vi "Stim prot to numeric array.vi"(9 "Calibration Key":string, 10 "Skip Pixel Mapping? (Same I/S Path)":bool, 11 "Stm Protocol":string[][](array[string])=[["1[73,55]", " 50u", " 50u", " 1", " 0", " 50u"], ["2[118,83]", " 50u", " 50u", " 1", " 0", " 50u"], ["3[102,121]", " 50u", " 50u", " 1", " 0", " 50u"], ["4[74,129]", " 50u", " 50u", " 1", " 0", " 50u"], ["5[83,156]", " 50u", " 50u", " 1", " 0", " 50u"]]) -> (1 "Stim Array (with voltage) OUT":T1[](array[typedef]))   [LabVIEW 2012]
uses:
  Custom Controls and Typedefs/Stim Waveform Parameters.ctl
  Custom Controls and Typedefs/Params for Galvo Voltage Calculation (Y Axis).ctl
  Custom Controls and Typedefs/Params for Galvo Voltage Calculation (X Axis).ctl
  GFG/GFG library.lvlib
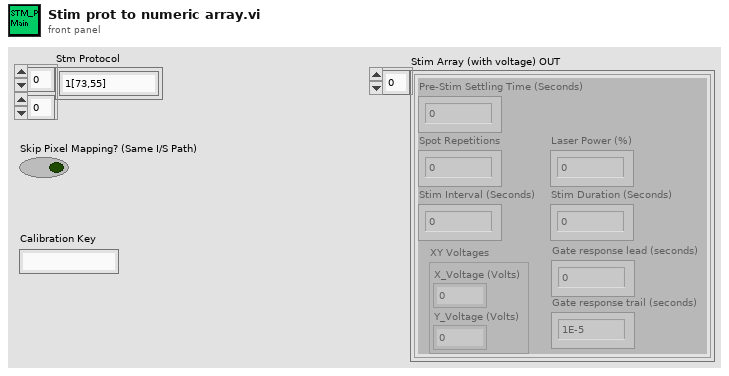
[diagram p1: front panel]
types:
  T1 = typedef "Stim Waveform Parameters.ctl" = cluster{"Stim Interval (Seconds)":dbl, "Pre-Stim Settling Time (Seconds)":dbl, "Stim Duration (Seconds)":dbl, "Spot Repetitions":i32, "Laser Power (%)":dbl, "XY Voltages":cluster{"X_Voltage (Volts)":dbl, "Y_Voltage (Volts)":dbl}, "Gate response lead (seconds)":dbl, "Gate response trail (seconds)":dbl}
  T2 = typedef "Params for Galvo Voltage Calculation (X Axis).ctl" = cluster{"X.Voltage(Max)":dbl, "X.Volt.Offset":dbl, "Tot.X.Pixels":u32, "X.Pixel.Index":u32}
  T3 = typedef "Params for Galvo Voltage Calculation (Y Axis).ctl" = cluster{"Y.Voltage(Max)":dbl, "Y.Volt.Offset":dbl, "Tot.Y.Pixels":u32, "Y.Pixel.Index":u32}
  T4 = typedef "Calibration Key Param structure.ctl" = cluster{"GFG Variable Name":string, "Data Type":T5, "Value":variant}
  T5 = typedef "VariantType.lvlib/Type.ctl" = enum8{"Invalid Type", "Void", "I8", "I16", "I32", "I64", "U8", "U16", "U32", "U64", "Single Float", "Double Float", "Extended Float", "Single Complex", "Double Complex", "Extended Complex", "Enum U8", "Enum U16", "Enum U32", "Enum U64", "Single Float With Unit", "Double Float With Unit", "Extended Float With Unit", "Single Complex with Unit", "Double Complex with Unit", "Extended Complex with Unit", "Boolean", "String", "Path", "Picture", "Tag", "Array", "Cluster", "Variant", "LV Variant", "Waveform", "Timestamp", "Digital Waveform", "Digital Data", "ExpressData", "Refnum", "External Data", "VI", "Poly VI", "LabVIEW Class Instance", "Fixed Point"}
  T6 = cluster{"X_Pixel_Voltage":dbl, "Y_Pixel_Voltage":dbl}
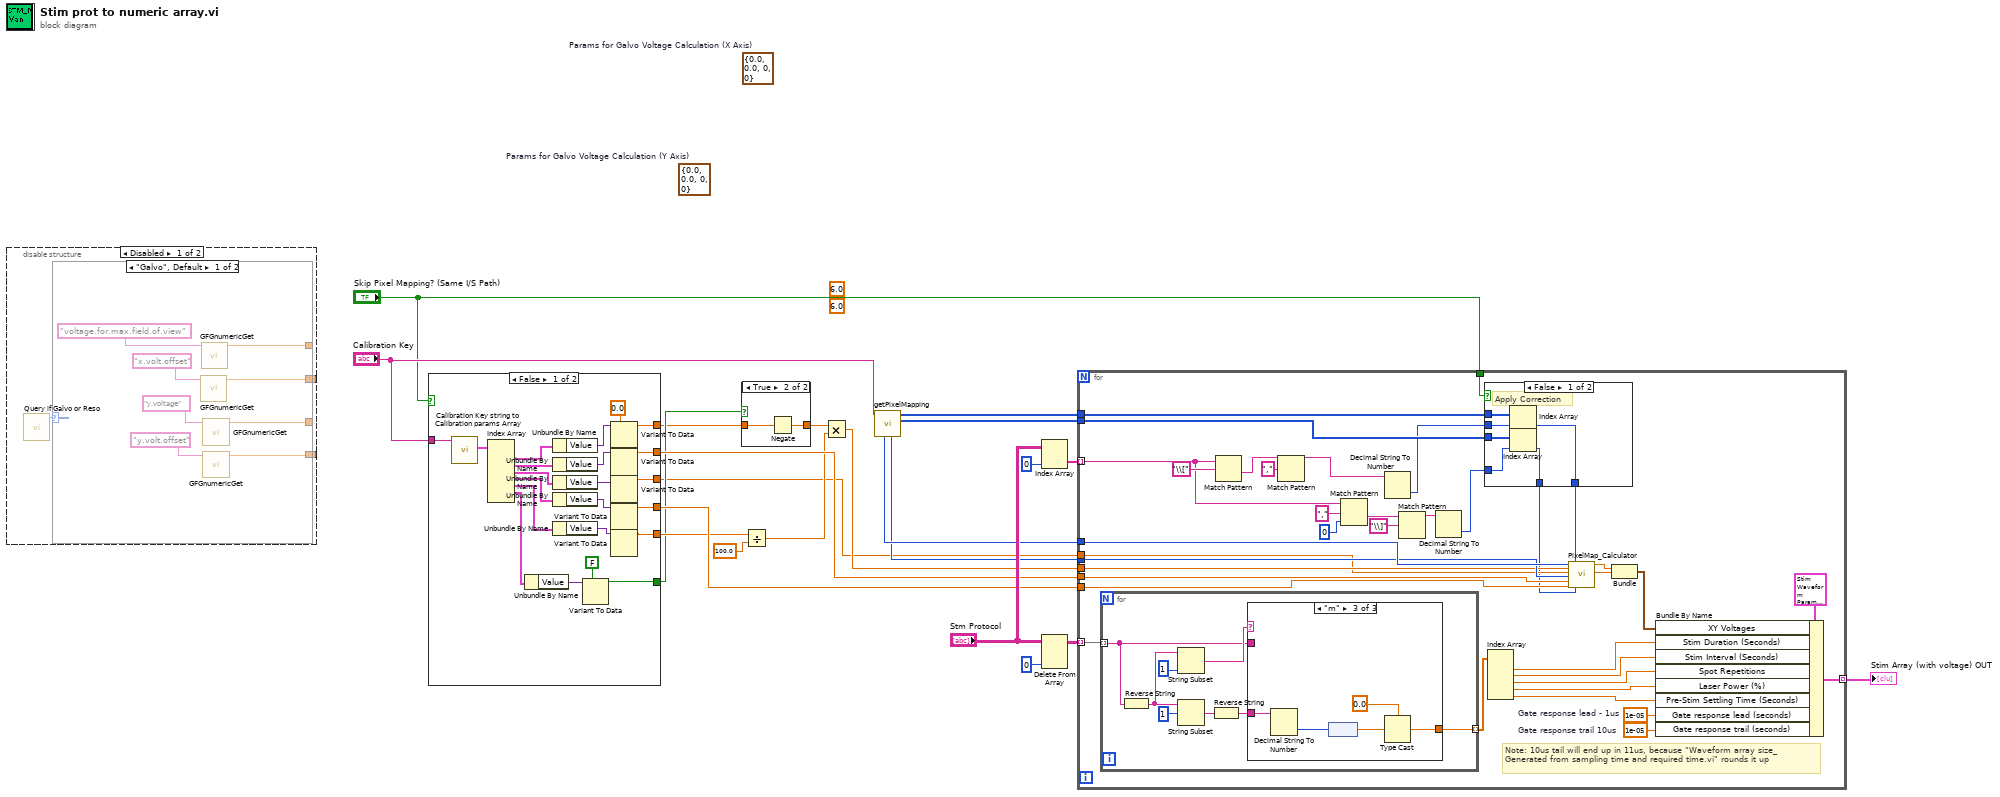
[diagram p0: block diagram]
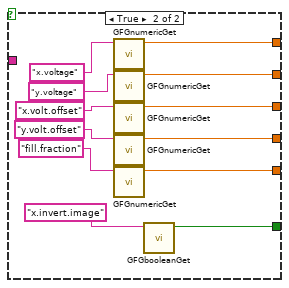
[diagram p3: hidden frame]
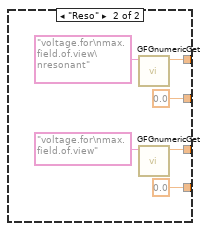
[diagram p4: hidden frame]
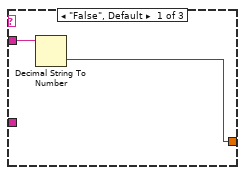
[diagram p7: hidden frame]
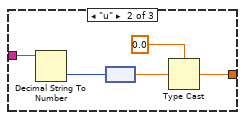
[diagram p8: hidden frame]
diagram:
  (unwired) T2 {"X.Voltage(Max)"=0.0, "X.Volt.Offset"=0.0, "Tot.X.Pixels"=0, "X.Pixel.Index"=0}  # Params for Galvo Voltage Calculation (X Axis)
  (unwired) T3 {"Y.Voltage(Max)"=0.0, "Y.Volt.Offset"=0.0, "Tot.Y.Pixels"=0, "Y.Pixel.Index"=0}  # Params for Galvo Voltage Calculation (Y Axis)
  (unwired) 6.0 ("Numeric")
  (unwired) 6.0 ("Numeric")
  n1 = disable-structure shown="Disabled" {
    disable-tunnel: [w24 _] -> _
    disable-tunnel: [w23 _] -> _
    frame Disabled {
      n2 = call "Query if Galvo or Reso.vi"() -> ("System Type"=w25:enum16{"Galvo", "Reso"})  [unwired: 10 in, 1 out]
      n3 = case shown="\"Galvo\", Default" w25 {
        tunnel: [w29 w37] -> _
        tunnel: [w28 0.0 ("Numeric")] -> w24
        tunnel: [w27 w36] -> _
        tunnel: [w26 0.0 ("Numeric")] -> w23
        frame "Galvo", Default {
          n4 = call "GFGnumericGet.vi"("Variable Name in"="x.volt.offset") -> ("Numeric"=w28:dbl)  [unwired: 8 in, 2 out]
          n5 = call "GFGnumericGet.vi"("Variable Name in"="voltage.for.max.field.of.view") -> ("Numeric"=w29:dbl)  [unwired: 8 in, 2 out]
          n6 = call "GFGnumericGet.vi"("Variable Name in"="y.voltage") -> ("Numeric"=w27:dbl)  [unwired: 8 in, 2 out]
          n7 = call "GFGnumericGet.vi"("Variable Name in"="y.volt.offset") -> ("Numeric"=w26:dbl)  [unwired: 8 in, 2 out]
        }
        frame "Reso" {
          n8 = call "GFGnumericGet.vi"("Variable Name in"="voltage.for\nmax.field.of.view\nresonant") -> ("Numeric"=w37:dbl)  [unwired: 8 in, 2 out]
          n9 = call "GFGnumericGet.vi"("Variable Name in"="voltage.for\nmax.field.of.view") -> ("Numeric"=w36:dbl)  [unwired: 8 in, 2 out]
        }
      }
    }
    frame Enabled {
    }
  }
  n10 = case shown="False" "Skip Pixel Mapping? (Same I/S Path)" {
    tunnel: "Calibration Key" -> [w61 _]
    tunnel: [w40 w66] -> w3
    tunnel: [w51 w67] -> w11
    tunnel: [w50 w65] -> w10
    tunnel: [w46 w64] -> w9
    tunnel: [w45 w68] -> w2
    tunnel: [w41 w62] -> w4
    frame False {
      w47 = 0.0
      n11 = call "Calibration Key string to Calibration params Array.vi"("Key String IN"=w61) -> ("Photostim Galvo Key Array"=w60:T4[])  [unwired: 8 in, 2 out]
      n12 = Index Array(array=w60) -> (element #1=w59:T4, element #2=w58:T4, element #3=w57:T4, element #4=w56:T4, element #5=w49:T4, element #6=w43:T4)  [unwired: 7 in, 1 out]
      n13 = Unbundle By Name(w43) -> ("Value"=w44:variant)
      n14 = Unbundle By Name(w59) -> ("Value"=w55:variant)
      n15 = Unbundle By Name(w58) -> ("Value"=w54:variant)
      n16 = Unbundle By Name(w57) -> ("Value"=w53:variant)
      n17 = Unbundle By Name(w56) -> ("Value"=w52:variant)
      n18 = Unbundle By Name(w49) -> ("Value"=w48:variant)
      n19 = Variant To Data(type=FALSE, Variant=w44) -> (data=w41:bool)  [unwired: 1 in, 1 out]
      n20 = Variant To Data(type=w47, Variant=w55) -> (data=w45:dbl)  [unwired: 1 in, 1 out]
      n21 = Variant To Data(type=w47, Variant=w54) -> (data=w51:dbl)  [unwired: 1 in, 1 out]
      n22 = Variant To Data(type=w47, Variant=w53) -> (data=w40:dbl)  [unwired: 1 in, 1 out]
      n23 = Variant To Data(type=w47, Variant=w52) -> (data=w50:dbl)  [unwired: 1 in, 1 out]
      n24 = Variant To Data(type=w47, Variant=w48) -> (data=w46:dbl)  [unwired: 1 in, 1 out]
    }
    frame True {
      n25 = call "GFGnumericGet.vi"("Variable Name in"="x.voltage") -> ("Numeric"=w68:dbl)  [unwired: 8 in, 2 out]
      n26 = call "GFGnumericGet.vi"("Variable Name in"="y.voltage") -> ("Numeric"=w67:dbl)  [unwired: 8 in, 2 out]
      n27 = call "GFGnumericGet.vi"("Variable Name in"="x.volt.offset") -> ("Numeric"=w66:dbl)  [unwired: 8 in, 2 out]
      n28 = call "GFGnumericGet.vi"("Variable Name in"="y.volt.offset") -> ("Numeric"=w65:dbl)  [unwired: 8 in, 2 out]
      n29 = call "GFGnumericGet.vi"("Variable Name in"="fill.fraction") -> ("Numeric"=w64:dbl)  [unwired: 8 in, 2 out]
      n30 = call "GFGbooleanGet.vi"("Variable Name in"="x.invert.image") -> ("Boolean Value OUT"=w62:bool)  [unwired: 9 in, 1 out]
    }
  }
  n31 = case shown="True" w4 {
    tunnel: w2 -> [w74 w76]
    tunnel: [w74 w75] -> w1
    frame False {
    }
    frame True {
      n32 = Negate(x=w76) -> (-x=w75:dbl)
    }
  }
  n33 = Divide(x=w9, y=100.0) -> (x/y=w7:dbl)
  n34 = Multiply(x=w1, y=w7) -> (x*y=w6:dbl)
  n35 = call "getPixelMapping.vi"("Key String IN"="Calibration Key") -> ("Y_Pixel Map"=w15:i32[], "X_Pixel Map"=w16:i32[], "y.pixels"=w13:i32, "x.pixels"=w14:i32)  [unwired: 5 in, 2 out]
  n36 = Index Array(array="Stm Protocol", index (col)=0 ("disabled index (col)")) -> (element=w18:string[])  [unwired: 1 in]
  n37 = Delete From Array(array="Stm Protocol", index (col)=0 ("disabled index (col)")) -> (array with subset deleted=w21:string[][])  [unwired: 2 in, 1 out]
  n38 = for {
    tunnel: w21 -> [w113] mode=indexing
    tunnel: w18 -> [w95] mode=indexing
    tunnel: [w100] -> w17 mode=indexing
    tunnel: w16 -> [w92]
    tunnel: w15 -> [w91]
    tunnel: w14 -> [w90]
    tunnel: w13 -> [w89]
    tunnel: w6 -> [w86]
    tunnel: w3 -> [w85]
    tunnel: w11 -> [w84]
    tunnel: w10 -> [w83]
    tunnel: "Skip Pixel Mapping? (Same I/S Path)" -> [w77]
    w78 = 1e-05  # Gate response trail 10us
    w79 = 1e-05  # Gate response lead - 1us
    # "Note: 10us tail will end up in 11us, because \"Waveform array size_Generated from sampling time and required time.vi\" rounds it up"
    n39 = for {
      tunnel: w113 -> [w122] mode=indexing
      tunnel: [w123] -> w107 mode=indexing
      n40 = Reverse String(1:w122) -> (0:w126:string)
      n41 = String Subset(string=w126, length (rest)=1 ("length (rest)")) -> (substring=w124:string)  [unwired: 1 in]
      n42 = String Subset(string=w126, offset (0)=1) -> (substring=w128:string)  [unwired: 1 in]
      n43 = Reverse String(1:w128) -> (0:w127:string)
      n44 = case shown="\"m\"" w124 {
        tunnel: w127 -> [_ w136 w141]
        tunnel: [w131 w132 w137] -> w123
        tunnel: w122 -> [w130 _ _]
        frame "False", Default {
          n45 = Decimal String To Number(string=w130) -> (number=w131:i32)  [unwired: 2 in, 1 out]
        }
        frame "u" {
          n46 = Decimal String To Number(string=w136) -> (number=w135:i32)  [unwired: 2 in, 1 out]
          n47 = node(w135) -> (w133:dbl[unit])
          n48 = Type Cast(type=0.0 ("stim duration (in seconds) 2"), x=w133) -> (*(type *) &x=w132:dbl)
        }
        frame "m" {
          n49 = Decimal String To Number(string=w141) -> (number=w140:i32)  [unwired: 2 in, 1 out]
          n50 = node(w140) -> (w138:dbl[unit])
          n51 = Type Cast(type=0.0 ("stim duration (in seconds) 2"), x=w138) -> (*(type *) &x=w137:dbl)
        }
      }
    }
    n52 = Match Pattern(string=w95, regular expression="\\[") -> (after substring=w99:string)  [unwired: 1 in, 3 out]
    n53 = Match Pattern(string=w99, regular expression=",") -> (before substring=w97:string)  [unwired: 1 in, 3 out]
    n54 = Match Pattern(string=w95, regular expression=",", offset (0)=0) -> (after substring=w110:string)  [unwired: 3 out]
    n55 = Decimal String To Number(string=w97) -> (number=w88:i32)  [unwired: 2 in, 1 out]
    n56 = Match Pattern(string=w110, regular expression="\\]") -> (before substring=w108:string)  [unwired: 1 in, 3 out]
    n57 = Decimal String To Number(string=w108) -> (number=w87:i32)  [unwired: 2 in, 1 out]
    n58 = case shown="False" w77 {
      tunnel: w92 -> [w119 _]
      tunnel: w91 -> [w118 _]
      tunnel: w88 -> [w117 w121]
      tunnel: w87 -> [w116 w120]
      tunnel: [w115 w121] -> w81
      tunnel: [w114 w120] -> w80
      frame False {
        # "Apply Correction"
        n59 = Index Array(array=w119, index=w117) -> (element=w115:i32)
        n60 = Index Array(array=w118, index=w116) -> (element=w114:i32)
      }
      frame True {
      }
    }
    n61 = Index Array(array=w107) -> (element #1=w105:dbl, element #2=w104:dbl, element #3=w103:dbl, element #4=w102:dbl, element #5=w101:dbl)  [unwired: 5 in]
    n62 = call "PixelMap_Calculator.vi"("Tot.X.Pixels"=w90, "X.Voltage(Max)"=w86, "X.Volt.Offset"=w85, "Tot.Y.Pixels"=w89, "Y.Voltage(Max)"=w84, "Y.Volt.Offset"=w83, "X.Pixel.Index"=w81, "Y.Pixel.Index"=w80) -> ("X_Pixel_Voltage"=w94:dbl, "Y_Pixel_Voltage"=w93:dbl)  [unwired: 10 in]
    n63 = Bundle("X_Pixel_Voltage"=w94, "Y_Pixel_Voltage"=w93) -> (w82:T6)  [unwired: 1 in]
    n64 = Bundle By Name(cluster=T1 {"Stim Interval (Seconds)"=0.0, "Pre-Stim Settling Time (Seconds)"=0.0, "Stim Duration (Seconds)"=0.0, "Spot Repetitions"=0, "Laser Power (%)"=0.0, "XY Voltages"={"X_Voltage (Volts)"=0.0, "Y_Voltage (Volts)"=0.0}, "Gate response lead (seconds)"=1e-06, "Gate response trail (seconds)"=0.0} ("Stim Waveform Parameters"), "XY Voltages"=w82, "Stim Duration (Seconds)"=w105, "Stim Interval (Seconds)"=w104, "Spot Repetitions"=w103, "Laser Power (%)"=w102, "Pre-Stim Settling Time (Seconds)"=w101, "Gate response lead (seconds)"=w79, "Gate response trail (seconds)"=w78) -> (w100:T1)
  }
  "Stim Array (with voltage) OUT" <- w17
